vi "Init_All_AE.vi"(7 "Flat File Path":path=path "C:/Users/STED/Desktop/Cambridge STED Control Software/Host VIs/SLM/Flatness Correction LSH0700935/CAL_LSH0700935_770nm.bmp", 8 "HoloArray In":T1[](array[typedef]) {"Modes"."Amplititute" step=0.05}, 11 "General settings":T2={"Holo size (pixels)"=300, "Top hat radius"=0.5, "Number of modes"=20, "Bkg gradient X"=-40.0, "Bkg gradient Y"=-40.0, "Flat"=FALSE, "Mode Matrix"=0}) -> (0 "Holo Array Out":T1[](array[typedef]) {"Modes"."Amplititute" step=0.05})   [LabVIEW 2014]
uses:
  Controls/Holo Settings.ctl
  Controls/SLM General Settings.ctl
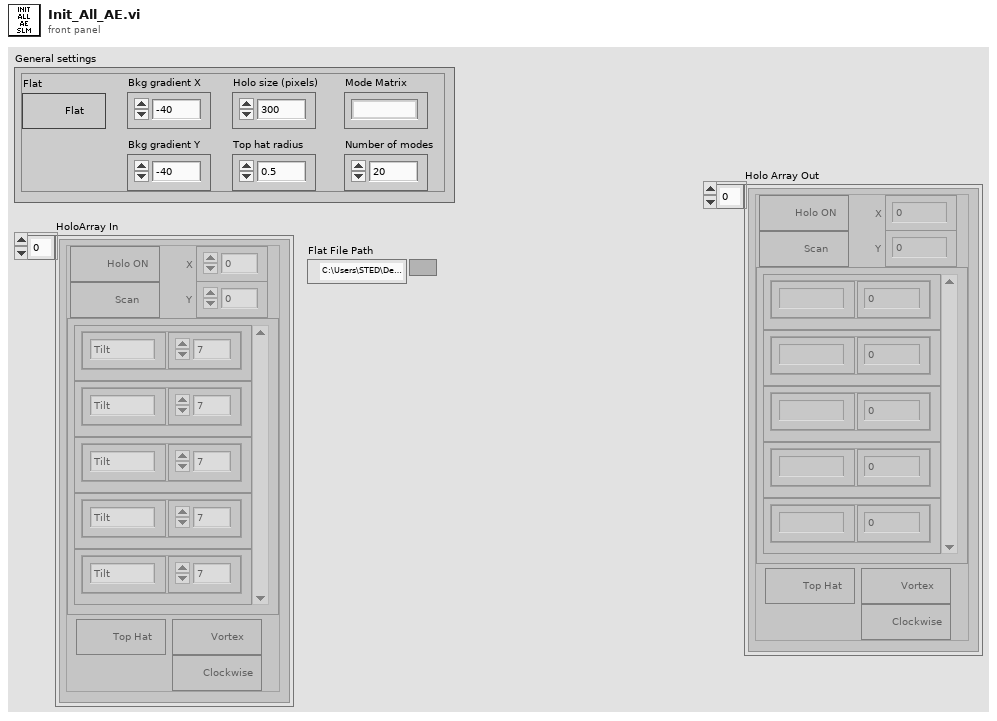
[diagram p1: front panel]
types:
  T1 = typedef "Holo Settings.ctl" = cluster{"Top Hat":bool, "Modes":cluster{"Mode ID":string, "Amplititute":dbl}[], "Vortex":bool, "Clockwise":bool, "X":dbl, "Y":dbl, "Holo ON":bool, "Scan":bool}
  T2 = typedef "SLM General Settings.ctl" = cluster{"Holo size (pixels)":i32, "Top hat radius":dbl, "Number of modes":i32, "Bkg gradient X":dbl, "Bkg gradient Y":dbl, "Flat":bool, "Mode Matrix":u16}
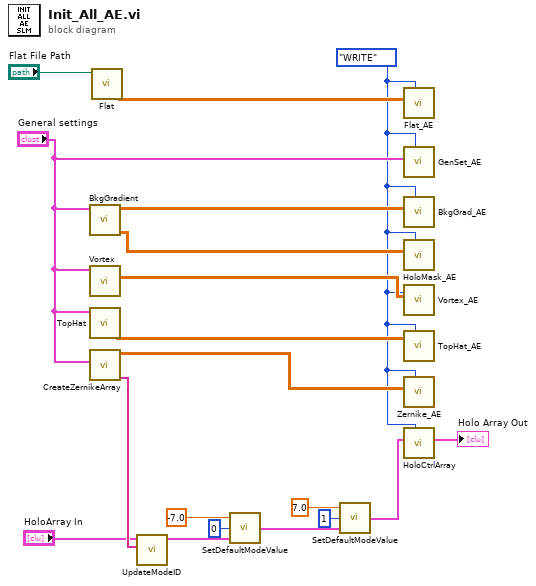
[diagram p0: block diagram]
diagram:
  w9 = enum16{"READ", "WRITE"}."WRITE" ("Action")
  n1 = call "BkgGradient.vi"("General settings"="General settings") -> ("Holo mask"=w12:dbl[][], "gradient"=w11:dbl[][])  [unwired: 9 in]
  n2 = call "Vortex.vi"("General settings"="General settings") -> ("Vortex"=w16:dbl[][])  [unwired: 10 in]
  n3 = call "TopHat.vi"("General settings"="General settings") -> ("TopHat"=w15:dbl[][])  [unwired: 10 in]
  n4 = call "CreateZernikeArray.vi"("General settings"="General settings") -> ("Mode IDs"=w13:string[], "Modes Out"=w14:dbl[][][])  [unwired: 9 in]
  n5 = call "Flat.vi"("File Path"="Flat File Path") -> ("Flatness"=w19:dbl[][])  [unwired: 10 in]
  n6 = call "UpdateModeID.vi"("Mode IDs"=w13, "Array in"="HoloArray In") -> ("Array out"=w8:T1[])  [unwired: 9 in]
  n7 = call "SetDefaultModeValue.vi"("Array in"=w8, "index"=0, "Amplititute"=-7.0) -> ("output array"=w5:T1[])
  n8 = call "SetDefaultModeValue.vi"("Array in"=w5, "index"=1, "Amplititute"=7.0) -> ("output array"=w2:T1[])
  n9 = call "Flat_AE.vi"("Action"=w9, "Flat In"=w19) -> ()  [unwired: 9 in, 1 out]
  n10 = call "GenSet_AE.vi"("Enum"=w9, "General settings"="General settings") -> ()  [unwired: 9 in, 1 out]
  n11 = call "BkgGrad_AE.vi"("Action"=w9, "BkgGrad In"=w11) -> ()  [unwired: 9 in, 1 out]
  n12 = call "HoloMask_AE.vi"("Action"=w9, "HoloMask In"=w12) -> ()  [unwired: 9 in, 1 out]
  n13 = call "Vortex_AE.vi"("Action"=w9, "Vortex In"=w16) -> ()  [unwired: 9 in, 1 out]
  n14 = call "TopHat_AE.vi"("Action"=w9, "TopHat In"=w15) -> ()  [unwired: 9 in, 1 out]
  n15 = call "Zernike_AE.vi"("Action"=w9, "Zernike In"=w14) -> ()  [unwired: 9 in, 1 out]
  n16 = call "HoloCtrlArray.vi"("Action"=w9, "Holo Array In"=w2) -> ("Holo Array Out"=→"Holo Array Out":T1[])  [unwired: 9 in]
